vi "Get SMO Public API.vi"(8 "error in (no error)":errorcluster, 11 "Instrument.Strain in":refnum<class "Instrument.Strain.lvclass">) -> (0 "error out":errorcluster, 2 "commands":string[](array[string]), 3 "Instrument.Strain out":refnum<class "Instrument.Strain.lvclass">)   [LabVIEW 2019, in "Instrument.Strain.lvclass"]
doc: "Override this VI to return a list of commands supported by your Instrument"
uses:
  Instrument.Strain.lvclass
  Typedefs/Strain.Commands--Enum.ctl
  bcf8792a-54ad-4a3e-88d6-091b5e09e2f5.vi
  <userlib>/LevyLab/Instrument Framework/Instrument/Instrument.lvclass
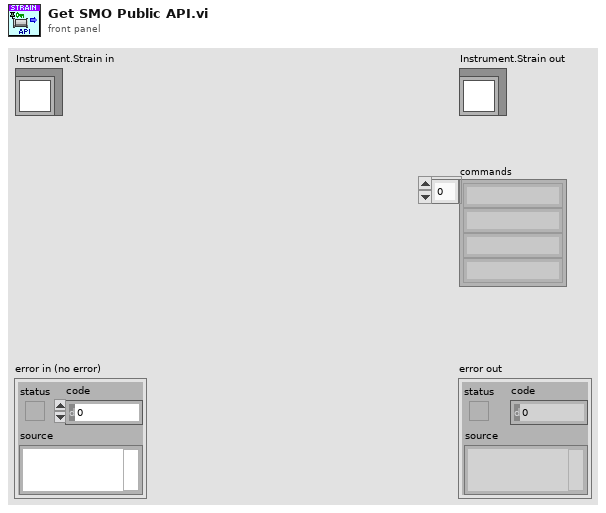
[diagram p1: front panel]
types:
  T1 = typedef "Instrument.Strain.lvclass/Strain.Commands--Enum.ctl" = enum16{"getStrain", "setStrain"}
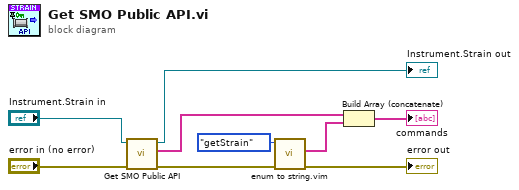
[diagram p0: block diagram]
diagram:
  n1 = call-parent "Get SMO Public API.vi"("error in (no error)"="error in (no error)", "Instrument in"="Instrument.Strain in") -> ("error out"=→"error out":errorcluster, "commands"=w2:string[], "Instrument out"=→"Instrument.Strain out":refnum<class "Instrument.Strain.lvclass">)  [unwired: 7 in]
  n2 = call "enum to string.vim"("enum in"=Strain.Commands--Enum."getStrain" ("Command")) -> ("strings out"=w1:string[])  [unwired: 9 in, 1 out]
  n3 = Build Array (concatenate)(w2, w1) -> (→"commands":string[])
